vi "Rhythm-Create.vi"(0 "Data in":T1, 9 "Npts":i32, 11 "error in (no error)":errorcluster) -> (4 "Data out":T1, 8 "Y":dbl[](array[numeric]), 15 "error out":errorcluster)   [LabVIEW 2020]
uses:
  Rhythm-Data.ctl
  <vilib>/Analysis/NI_AALBase.lvlib
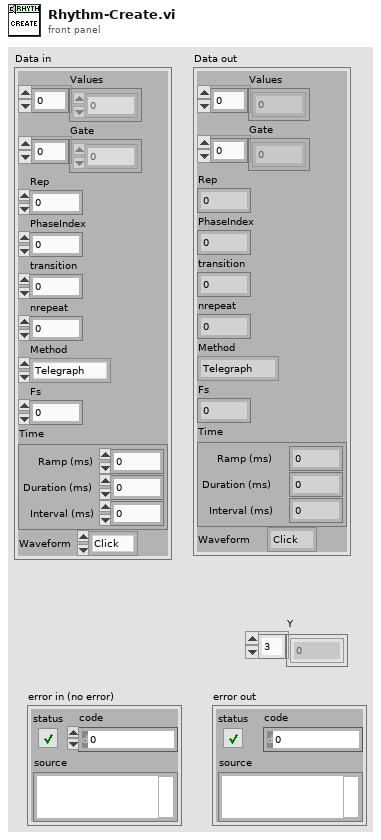
[diagram p1: front panel]
types:
  T1 = typedef "Rhythm-Data.ctl" = cluster{"Values":dbl[], "Gate":dbl[], "Rep":i32, "PhaseIndex":i32, "transition":i32, "nrepeat":i32, "Method":enum16{"Telegraph", "Interval"}, "Fs":dbl, "Time":cluster{"Ramp (ms)":dbl, "Duration (ms)":dbl, "Interval (ms)":dbl}, "Waveform":enum16{"Click", "Noise"}}
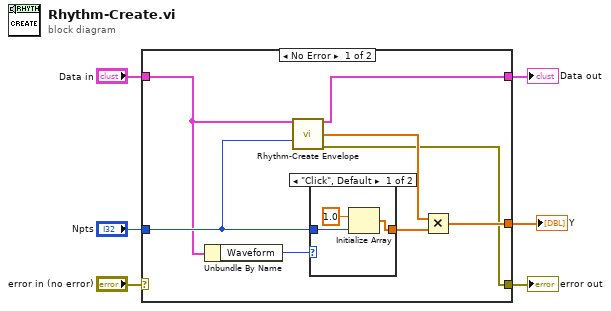
[diagram p0: block diagram]
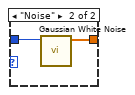
[diagram p2: hidden frame]
diagram:
  n1 = case shown="No Error" "error in (no error)" {
    selector: "error in (no error)" -> [_ w21]
    tunnel: "Data in" -> [w8 w20]
    tunnel: [w11 w20] -> w4
    tunnel: [w9 w21] -> w5
    tunnel: "Npts" -> [w12 _]
    tunnel: [w10 _] -> w1
    frame No Error {
      n2 = Unbundle By Name(w8) -> ("Waveform"=w7:enum16{"Click", "Noise"})
      n3 = call "Rhythm-Create Envelope.vi"("Data in"=w8, "Npts"=w12) -> ("Data out"=w11:T1, "Y"=w13:dbl[], "error out"=w9:errorcluster)  [unwired: 11 in]
      n4 = case shown="\"Click\", Default" w7 {
        tunnel: [w16 w19] -> w14
        tunnel: w12 -> [w17 w18]
        frame "Click", Default {
          n5 = Initialize Array(1.0 ("element"), w17) -> (w16:dbl[])
        }
        frame "Noise" {
          n6 = call <vilib>:"Gaussian White Noise.vi"("samples"=w18) -> ("Gaussian noise pattern"=w19:dbl[])  [unwired: 9 in, 1 out]
        }
      }
      n7 = Multiply(x=w13, y=w14) -> (x*y=w10:dbl[])
    }
    frame Error {
    }
  }
  "error out" <- w5
  "Data out" <- w4
  "Y" <- w1
